vi "2motor.vi"(0 "motor number 1":u8, 2 "name of motor group":string="RobotDrive", 5 "motor number 1":string="My Motor RefNum", 7 "secondsFromNeutralToFull":dbl, 9 "motor number 2":string="My Motor RefNum", 11 "motor number 2":u8) -> ()   [LabVIEW 2017]
uses:
  <vilib>/Rock Robotics/WPI/ThirdParty/Phoenix-LabVIEW/Motor Controller/Controls/CTRE_Phoenix_MotorControl_NeutralMode.ctl
  <vilib>/Rock Robotics/WPI/RobotDrive/WPI_RobotDriveOpen2MotorWithExistingMotors.vi
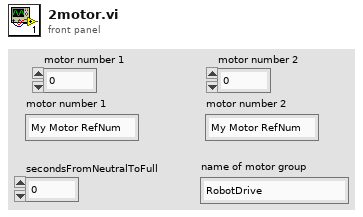
[diagram p1: front panel]
types:
  T1 = typedef "CTRE_Phoenix_MotorControl_NeutralMode.ctl" = enum8{"EEPROMSetting", "Override to Coast", "Override to Brake"}
  T2 = typedef "WPI_MotorControlDeviceRef.ctl" = cluster{"DeviceStatus":errorcluster, "Type":T3, "PWM":cluster{"PWM Channel":T4, "DeadBand":T5}, "CAN":cluster{"Device Number":u8, "SetOutput VI Ref":variant, "GetOutput VI Ref":variant, "Enable VI Ref":variant, "Disable VI Ref":variant, "Data":variant}, "Invert":bool, "DIO PWM":cluster{"PWM \"Enable\" Channel":T4, "DIOChannel":T6, "PWM Rate":dbl}}
  T3 = typedef "WPI_MotorControlType.ctl" = enum16{"PWM", "CAN", "DIO PWM"}
  T4 = typedef "FPGA_DIOPWMChannel.ctl" = enum8{"PWM 0", "PWM 1", "PWM 2", "PWM 3", "PWM 4", "PWM 5", "PWM 6", "PWM 7", "PWM 8", "PWM 9", "PWM MXP 0", "PWM MXP 1", "PWM MXP 2", "PWM MXP 3", "PWM MXP 4", "PWM MXP 5", "PWM MXP 6", "PWM MXP 7", "PWM MXP 8", "PWM MXP 9", "Invalid"}
  T5 = typedef "WPI_PWMDeadband.ctl" = cluster{"Name":string, "maxPositivePwm":i32, "minPositivePwm":i32, "centerPwm":i32, "maxNegativePwm":i32, "minNegativePwm":i32, "angularRange":u16}
  T6 = typedef "FPGA_DIOChannel.ctl" = enum8{"DIO 0", "DIO 1", "DIO 2", "DIO 3", "DIO 4", "DIO 5", "DIO 6", "DIO 7", "DIO 8", "DIO 9", "DIO MXP 0", "DIO MXP 1", "DIO MXP 2", "DIO MXP 3", "DIO MXP 4", "DIO MXP 5", "DIO MXP 6", "DIO MXP 7", "DIO MXP 8", "DIO MXP 9", "DIO MXP 10", "DIO MXP 11", "DIO MXP 12", "DIO MXP 13", "DIO MXP 14", "DIO MXP 15", "SPI Port CS1", "SPI Port CS2", "SPI Port CS3", "SPI Port MISO", "SPI Port MOSI", "Invalid"}
  T7 = typedef "WPI_RobotDriveDevRef.ctl" = cluster{"DevStatus":errorcluster, "Motors[]":T2[], "Square Inputs":bool, "Max Output":dbl}
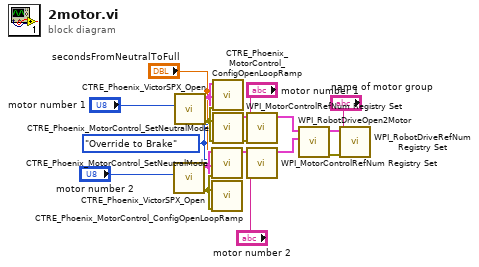
[diagram p0: block diagram]
diagram:
  w7 = CTRE_Phoenix_MotorControl_NeutralMode."Override to Brake" ("Motor Control Neutral Mode")
  n1 = call <vilib>:"CTRE_Phoenix_VictorSPX_Open.vi"("Device Number"="motor number 2") -> ("error out"=w14:errorcluster, "CAN Talon SRX Ref"=w13:T2)  [unwired: 9 in]
  n2 = call <vilib>:"CTRE_Phoenix_VictorSPX_Open.vi"("Device Number"="motor number 1") -> ("error out"=w18:errorcluster, "CAN Talon SRX Ref"=w17:T2)  [unwired: 9 in]
  n3 = call <vilib>:"CTRE_Phoenix_MotorControl_SetNeutralMode.vi"("error in (no error)"=w14, "Motor Control Neutral Mode"=w7, "PhoenixMotorControlDevRef"=w13) -> ("PhoenixMotorControlDevRef"=w12:T2)  [unwired: 7 in, 1 out]
  n4 = call <vilib>:"CTRE_Phoenix_MotorControl_ConfigOpenLoopRamp.vi"("error in (no error)"=w14, "secondsFromNeutralToFull"="secondsFromNeutralToFull", "PhoenixMotorControlDevRef"=w13) -> ()  [unwired: 7 in, 2 out]
  n5 = call <vilib>:"CTRE_Phoenix_MotorControl_ConfigOpenLoopRamp.vi"("error in (no error)"=w18, "secondsFromNeutralToFull"="secondsFromNeutralToFull", "PhoenixMotorControlDevRef"=w17) -> ()  [unwired: 7 in, 2 out]
  n6 = call <vilib>:"CTRE_Phoenix_MotorControl_SetNeutralMode.vi"("error in (no error)"=w18, "Motor Control Neutral Mode"=w7, "PhoenixMotorControlDevRef"=w17) -> ("error out"=w16:errorcluster, "PhoenixMotorControlDevRef"=w15:T2)  [unwired: 7 in]
  n7 = call <vilib>:"WPI_MotorControlRefNum Registry Set.vi"("error in (no error)"=w16, "refnum name"="motor number 1", "MotorControlDevRef"=w15) -> ("MotorControlDevRef"=w10:T2)  [unwired: 7 in, 1 out]
  n8 = call <vilib>:"WPI_MotorControlRefNum Registry Set.vi"("refnum name"="motor number 2", "MotorControlDevRef"=w12) -> ("MotorControlDevRef"=w11:T2)  [unwired: 8 in, 1 out]
  n9 = call-poly <vilib>:"WPI_RobotDriveOpen2Motor.vi"("Right Motor Dev Ref"=w11, "Left Motor Dev Ref"=w10) -> ("error out"=w8:errorcluster, "RobotDriveDevRef"=w9:T7)  [unwired: 8 in]
  n10 = call <vilib>:"WPI_RobotDriveRefNum Registry Set.vi"("error in (no error)"=w8, "refnum name"="name of motor group", "RobotDriveDevRef"=w9) -> ()  [unwired: 7 in, 2 out]
